vi "Average Images.vi"(0 "Array of Images":T1[](array[typedef]), 2 "Avg Image":T1, 5 "error in":errorcluster) -> (19 "error out":errorcluster)   [LabVIEW 2012]
doc: "Functional Global for the average Images of Group 1 and 2. Images will store the average images as a SGL image for sequence being run during the current iteration."
uses:
  <vilib>/vision/Image Controls.llb/IMAQ Image.ctl
  <vilib>/vision/NI_Vision_Development_Module.lvlib
panel:
  out "Array":T1[](array[plugin-control])
  out "Image":T1(plugin-control)
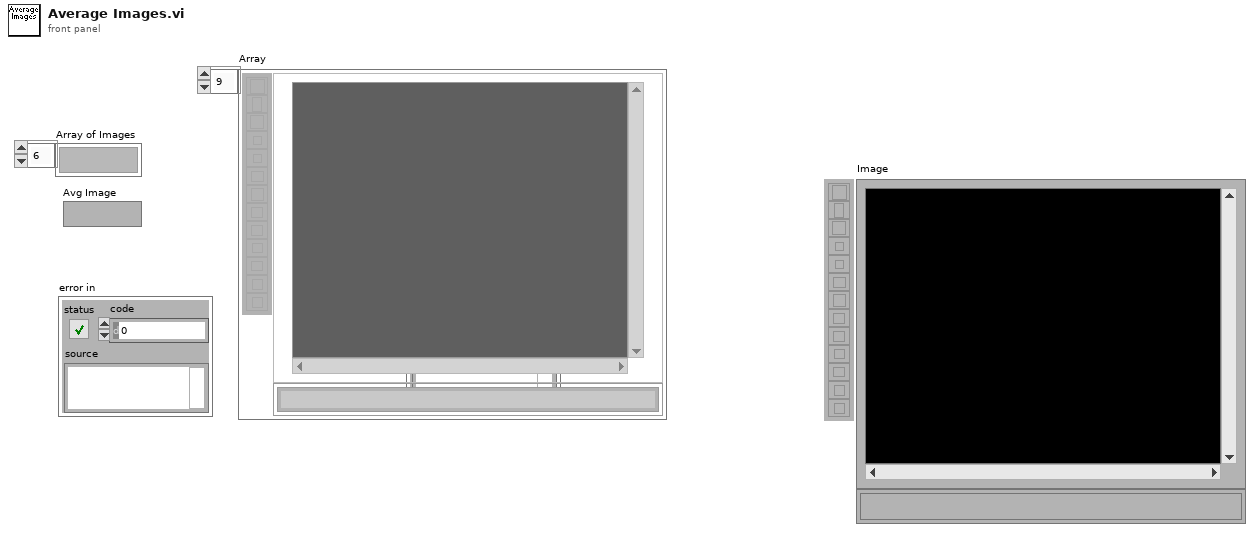
[diagram p1: front panel]
types:
  T1 = typedef "IMAQ Image.ctl" = refnum<image>
  T2 = typedef "Image Type" = u32
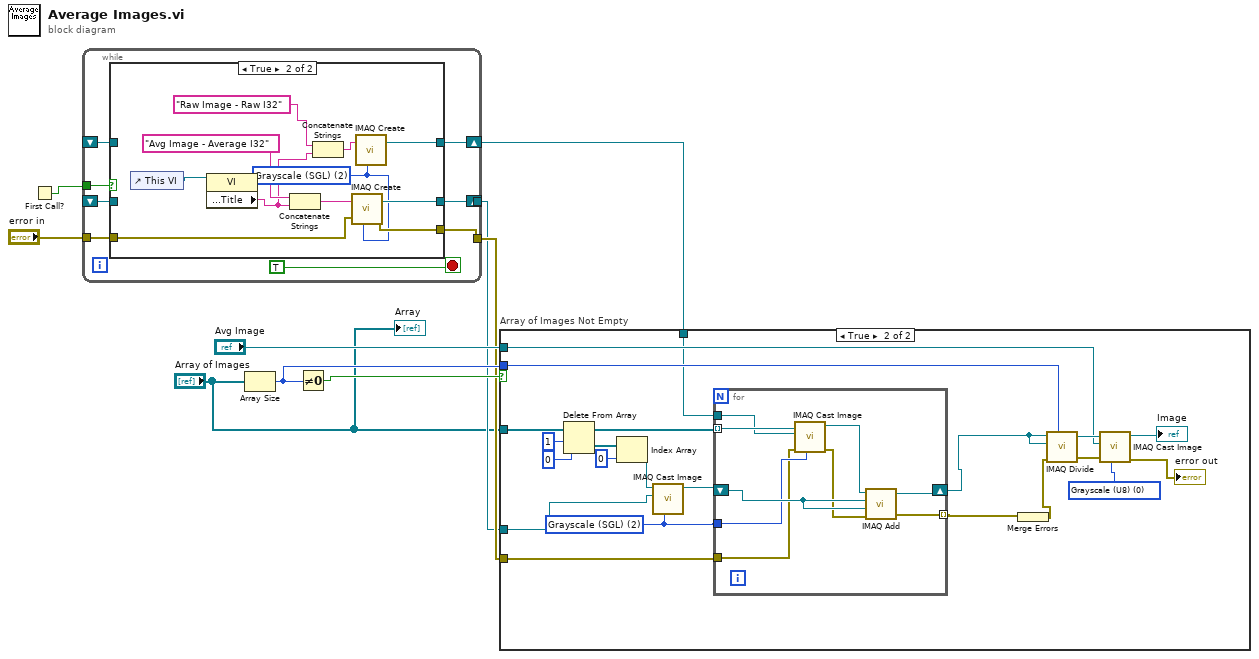
[diagram p0: block diagram]
diagram:
  n1 = First Call?() -> (First Call?: T/F=w6:bool)
  n2 = while {
    tunnel: w6 -> [w17]
    shift-right: [w12] -> w3
    shift-left: _ -> [w15]
    tunnel: "error in" -> [w14]
    tunnel: [w13] -> w4
    tunnel: [w12] -> _
    shift-right: [w11] -> w2
    shift-left: _ -> [w10]
    stop <- TRUE stop-if-true
    n3 = case shown="True" w17 {
      tunnel: [w20 w28] -> w12
      tunnel: w15 -> [w20 _]
      tunnel: w14 -> [w19 w27]
      tunnel: [w19 w26] -> w13
      tunnel: [w18 w22] -> w11
      tunnel: w10 -> [w18 _]
      frame False {
      }
      frame True {
        w21 = T2 2 items=["Grayscale (U8)", "Grayscale (I16)", "Grayscale (SGL)", "Complex (CSG)", "RGB (U32)", "HSL (U32)", "RGB (U64)", "Grayscale (U16)"] ("Image Type")
        n4 = control-ref of="This VI"() -> (w31:refnum<vi>)
        n5 = property class="VI"(reference=w31) -> ("Front Panel.Title"=w24:string)  [unwired: 1 in, 2 out]
        n6 = Concatenate Strings("Avg Image - Average I32" ("string"), w24) -> (w29:string)
        n7 = Concatenate Strings("Raw Image - Raw I32" ("string"), w24) -> (w25:string)
        n8 = call "IMAQ Create"("Image Name"=w29, "Image Type"=w21, "error in (no error)"=w27) -> ("New Image"=w28:T1, "error out"=w26:errorcluster)  [unwired: 2 in]
        n9 = call "IMAQ Create"("Image Name"=w25, "Image Type"=w21) -> ("New Image"=w22:T1)  [unwired: 3 in, 1 out]
      }
    }
  }
  n10 = Array Size(array="Array of Images") -> (size(s)=w7:i32)
  n11 = Not Equal To 0?(x=w7) -> (x != 0?=w9:bool)
  n12 = case "Array of Images Not Empty" shown="True" w9 {
    tunnel: "Array of Images" -> [_ w51]
    tunnel: "Avg Image" -> [_ w45]
    tunnel: w7 -> [_ w47]
    tunnel: w4 -> [_ w35]
    tunnel: w3 -> [_ w39]
    tunnel: w2 -> [_ w32]
    frame False {
    }
    frame True {
      w44 = T2 0 items=["Grayscale (U8)", "Grayscale (I16)", "Grayscale (SGL)", "Complex (CSG)", "RGB (U32)", "HSL (U32)", "RGB (U64)", "Grayscale (U16)"] ("Image Type")
      w36 = T2 2 items=["Grayscale (U8)", "Grayscale (I16)", "Grayscale (SGL)", "Complex (CSG)", "RGB (U32)", "HSL (U32)", "RGB (U64)", "Grayscale (U16)"] ("Image Type")
      n13 = Delete From Array(array=w51, length=1, index=0) -> (deleted portion=w50:T1[], array with subset deleted=w38:T1[])
      n14 = Index Array(array=w50, index=0) -> (element=w49:T1)
      n15 = call "IMAQ Cast Image"("Image Type"=w36, "Image Dst"=w39, "Image Src"=w49) -> ("Image Dst Out"=w37:T1)  [unwired: 7 in, 1 out]
      n16 = for {
        shift-right: [w57] -> w33
        shift-left: w37 -> [w61]
        tunnel: [w62] -> w34 mode=indexing
        tunnel: w38 -> [w59] mode=indexing
        tunnel: w36 -> [w58]
        tunnel: w35 -> [w56]
        tunnel: w32 -> [w54]
        n17 = call "IMAQ Cast Image"("Image Type"=w58, "error in (no error)"=w56, "Image Dst"=w54, "Image Src"=w59) -> ("error out"=w55:errorcluster, "Image Dst Out"=w60:T1)  [unwired: 6 in]
        n18 = call "IMAQ Add"("Image Src A"=w60, "Image Dst"=w61, "Image Src B"=w61, "error in (no error)"=w55) -> ("Image Dst Out"=w57:T1, "error out"=w62:errorcluster)  [unwired: 3 in]
      }
      n19 = Merge Errors(w34) -> (w42:errorcluster)
      n20 = call "IMAQ Divide"("Image Src A"=w33, "Constant"=w47, "Image Dst"=w33, "error in (no error)"=w42) -> ("Image Dst Out"=w46:T1, "error out"=w41:errorcluster)  [unwired: 3 in]
      n21 = call "IMAQ Cast Image"("Image Type"=w44, "error in (no error)"=w41, "Image Dst"=w45, "Image Src"=w46) -> ("error out"=→"error out":errorcluster, "Image Dst Out"=→"Image":T1)  [unwired: 6 in]
    }
  }
  "Array" <- "Array of Images"
